vi "Function.vi"(8 "error in (no error)":errorcluster, 10 "String A":string, 11 "One Terminal in":refnum<class "ToUpper_STR.lvclass">) -> (0 "error out":errorcluster, 2 "String":string, 3 "One Terminal out":refnum<class "ToUpper_STR.lvclass">)   [LabVIEW 2021, in "ToUpper_STR.lvclass"]
uses:
  ToUpper_STR.lvclass
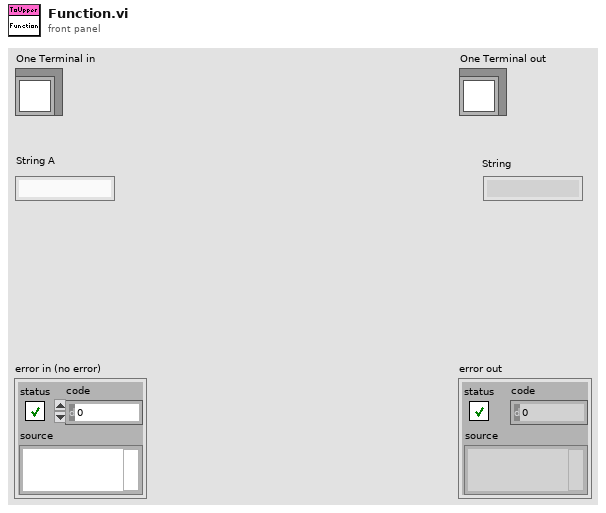
[diagram p1: front panel]
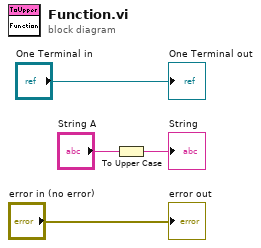
[diagram p0: block diagram]
diagram:
  n1 = To Upper Case(1:"String A") -> (0:→"String":string)
  "error out" <- "error in (no error)"
  "One Terminal out" <- "One Terminal in"
